vi "Error Test Start Bit Value.vi"(6 "error text in":string, 8 "error in":errorcluster, 9 "direction":string, 10 "start bit":i32) -> (0 "error out":errorcluster)   [LabVIEW 2020, in "ARINC 429 Import.lvlib"]
uses:
  ARINC 429 Import.lvlib
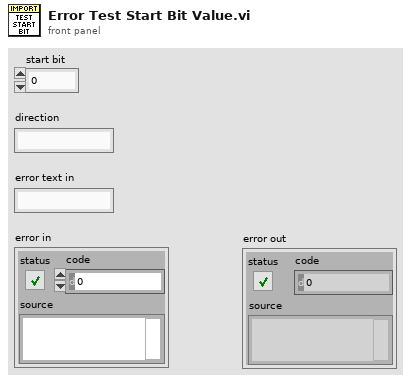
[diagram p1: front panel]
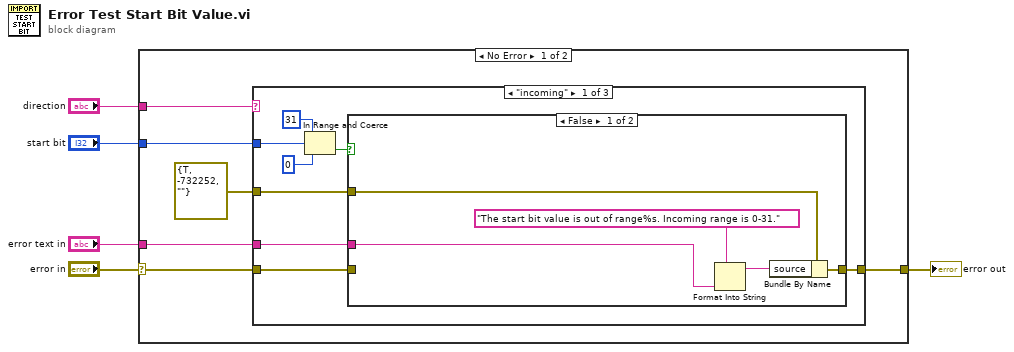
[diagram p0: block diagram]
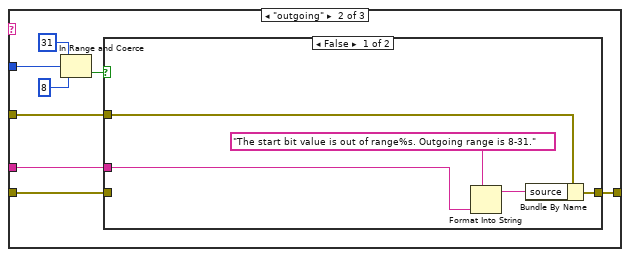
[diagram p3: hidden frame]
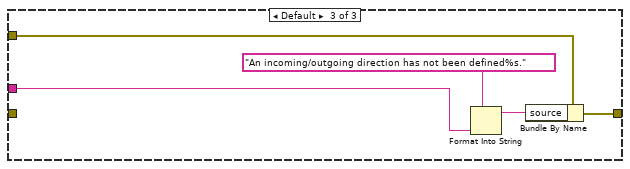
[diagram p5: hidden frame]
diagram:
  n1 = case shown="No Error" "error in" {
    selector: "error in" -> [w10 w45]
    tunnel: [w9 w45] -> w4
    tunnel: "start bit" -> [w11 _]
    tunnel: "direction" -> [w7 _]
    tunnel: "error text in" -> [w6 _]
    frame No Error {
      n2 = case shown="\"incoming\"" w7 {
        tunnel: errorcluster {"status"=TRUE, "code"=-732252, "source"=""} ("error constant") -> [w17 w31 w43]
        tunnel: [w18 w32 w44] -> w9
        tunnel: w11 -> [w14 w28 _]
        tunnel: w10 -> [w19 w33 _]
        tunnel: w6 -> [w12 w26 w42]
        frame "incoming" {
          n3 = In Range and Coerce(upper limit=31 ("lower limit"), x=w14, lower limit=0) -> (In Range?=w13:bool)  [unwired: 1 out]
          n4 = case shown="False" w13 {
            tunnel: w19 -> [_ w25]
            tunnel: [w23 w25] -> w18
            tunnel: w17 -> [w24 _]
            tunnel: w12 -> [w20 _]
            frame False {
              n5 = Format Into String(format string="The start bit value is out of range%s. Incoming range is 0-31." ("source"), w20) -> (resulting string=w22:string)  [unwired: 2 in, 1 out]
              n6 = Bundle By Name(cluster=w24, "source"=w22) -> (w23:errorcluster)
            }
            frame True {
            }
          }
        }
        frame "outgoing" {
          n7 = In Range and Coerce(upper limit=31 ("lower limit"), x=w28, lower limit=8) -> (In Range?=w27:bool)  [unwired: 1 out]
          n8 = case shown="False" w27 {
            tunnel: w33 -> [_ w39]
            tunnel: [w37 w39] -> w32
            tunnel: w31 -> [w38 _]
            tunnel: w26 -> [w34 _]
            frame False {
              n9 = Format Into String(format string="The start bit value is out of range%s. Outgoing range is 8-31." ("source"), w34) -> (resulting string=w36:string)  [unwired: 2 in, 1 out]
              n10 = Bundle By Name(cluster=w38, "source"=w36) -> (w37:errorcluster)
            }
            frame True {
            }
          }
        }
        frame Default {
          n11 = Format Into String(format string="An incoming/outgoing direction has not been defined%s." ("source"), w42) -> (resulting string=w41:string)  [unwired: 2 in, 1 out]
          n12 = Bundle By Name(cluster=w43, "source"=w41) -> (w44:errorcluster)
        }
      }
    }
    frame Error {
    }
  }
  "error out" <- w4
